vi "Fcurve sorted.vi"(8 "error in":errorcluster, 10 "Reply Payload":T1={"Fcurve out"=[], "Metadata out"={"dt (us)"=2.0, "Dec Factor"=1.0, "Z piezo Sensitivity (nm/V)"=6000.0, "K (N/m)"=0.6, "Sp (V)"=16.0, "Contact (ms)"=0.0, "Zpos contact"=2.000001, "Vel_app (nm/s)"=10000.0, "Vel_ret (nm/s)"=100000.0, "deltaV (nm)"=600.0, "Def_V0 (v)"=-0.113287, "Piezo gain"=1.0, "invOLS (nm/V)"=23.8}, "error"={"status"=FALSE, "code"=0, "source"=""}}) -> (0 "error out":errorcluster)   [LabVIEW 2019, in "Analysis.lvlib"]
doc: "_____\nCreated using DQMH Event Scripter 6.1.0.128."
uses:
  Analysis.lvlib
  Open Fcurve object (Reply Payload)--cluster.ctl
  Neo-Laura-LVOOP/Class Library/Fcurve_class/Metadata.ctl
  Neo-Laura-LVOOP/Class Library/Fcurve_class/Fcurve.lvclass
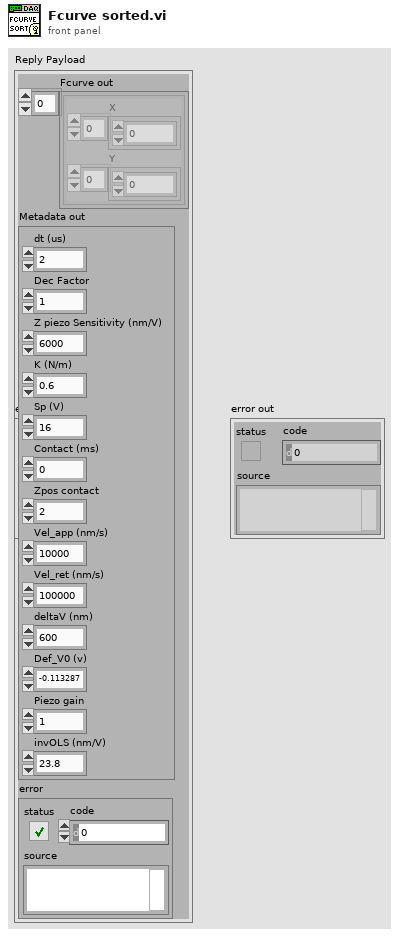
[diagram p1: front panel]
types:
  T1 = typedef "Analysis.lvlib/Open Fcurve object (Reply Payload)--cluster.ctl" = cluster{"Fcurve out":cluster{"X":dbl[], "Y":dbl[]}[], "Metadata out":T2, "error":errorcluster}
  T2 = typedef "Fcurve.lvclass/Metadata.ctl" = cluster{"dt (us)":dbl, "Dec Factor":dbl, "Z piezo Sensitivity (nm/V)":dbl, "K (N/m)":dbl, "Sp (V)":dbl, "Contact (ms)":dbl, "Zpos contact":dbl, "Vel_app (nm/s)":dbl, "Vel_ret (nm/s)":dbl, "deltaV (nm)":dbl, "Def_V0 (v)":dbl, "Piezo gain":dbl, "invOLS (nm/V)":dbl}
  T3 = typedef "Analysis.lvlib/Broadcast Events--cluster.ctl" = cluster{"Module Did Init":refnum<user-event>, "Status Updated":refnum<user-event>, "Error Reported":refnum<user-event>, "Module Did Stop":refnum<user-event>, "Update Module Execution Status":refnum<user-event>, "Fcurve sorted":refnum<user-event>}
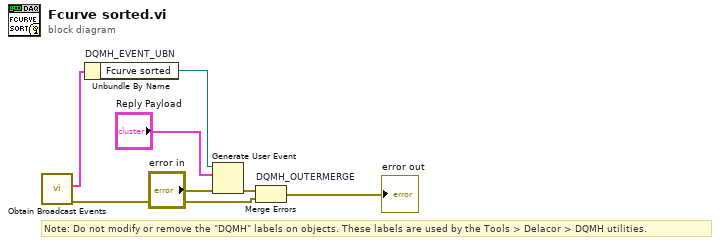
[diagram p0: block diagram]
diagram:
  # "Note: Do not modify or remove the \"DQMH\" labels on objects. These labels are used by the Tools > Delacor > DQMH utilities."
  n1 = call "Obtain Broadcast Events.vi"() -> ("error out"=w2:errorcluster, "Analysis Broadcast Events"=w1:T3)  [unwired: 10 in]
  n2 = Unbundle By Name "DQMH_EVENT_UBN"(w1) -> ("Fcurve sorted"=w4:refnum<user-event>)
  n3 = Generate User Event(user event=w4, event data cluster="Reply Payload", error in="error in") -> (error out=w3:errorcluster)  [unwired: 1 in, 1 out]
  n4 = Merge Errors "DQMH_OUTERMERGE"(w3, w2) -> (→"error out":errorcluster)
